vi "Publish Fast.vi"(8 "error in (no error)":errorcluster, 11 "RootModelPublishesUnthrottled in":refnum<class "ModelPublishesIndexA.lvclass">) -> (0 "error out":errorcluster, 3 "RootModelPublishesUnthrottled out":refnum<class "ModelPublishesIndexA.lvclass">)   [LabVIEW 2017, in "BenchmarkObservationRate.lvlib" / "ModelPublishesIndexA.lvclass"]
uses:
  ModelPublishesIndexA.lvclass
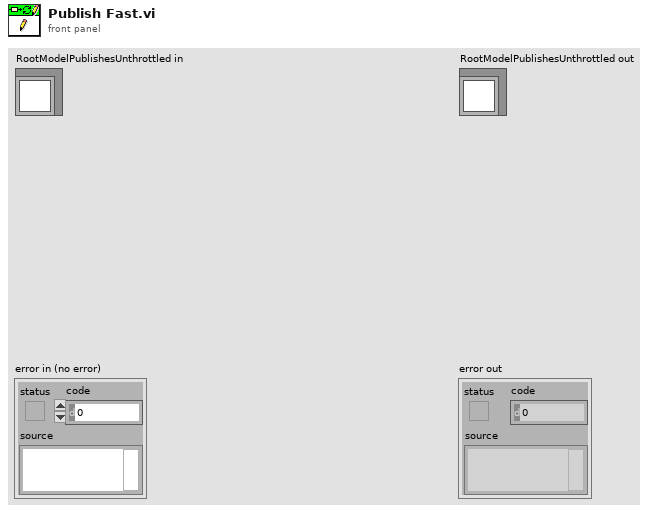
[diagram p1: front panel]
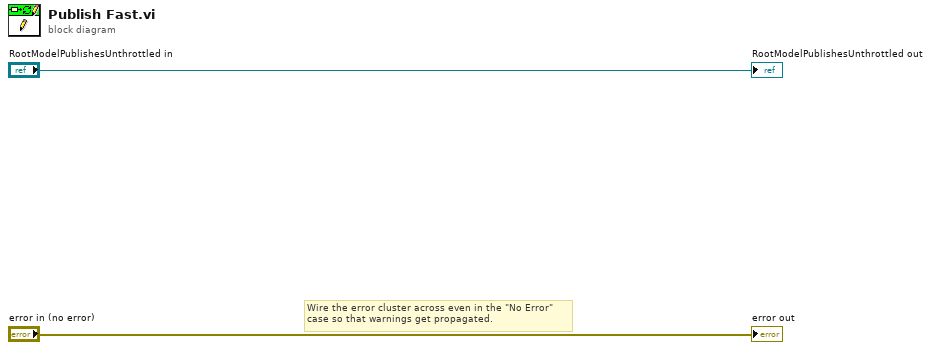
[diagram p0: block diagram]
diagram:
  # "Wire the error cluster across even in the \"No Error\"\ncase so that warnings get propagated."
  "error out" <- "error in (no error)"
  "RootModelPublishesUnthrottled out" <- "RootModelPublishesUnthrottled in"
